vi "SPADQ_GetData.vi"(7 "DelayCorrect?":bool, 8 "error in (no error)":errorcluster, 11 "Digitizer Settings":T1 {"Trigger Settings"."Trig Slope" items=["Positive", "Negative"]; "Trigger Settings"."Level (mV)" format="%.2f"; "Trigger Settings"."Trig Coupling" items=["DC 1 MOhm", "AC 1 MOhm", "DC 50 Ohm", "AC 50 Ohm"]; "Trigger Settings"."Trig Source" items=["Chan 1", "External"]; "Rel Dig Delay" format="%.2f"; "DigTimeOut" format="%.2f"; "Avg Num" min=1; "Offset delay (us)" format="%.2f"; "Additional dig delay (us)" format="%.2f"; "Digitizer delay (us)" format="%.2f"}) -> (0 "error out":errorcluster, 1 "Data Out":i16[][](array[numeric]), 3 "ADQAPI Ref (out)":refnum<k24>)   [LabVIEW 2022 SP3]
doc: "_____AlazarTech, Scope_____\n\nSet the Trigger delay"
uses:
  C:/Windows/System32/ADQAPI_dotNet_helper.dll
  -DigitizerRoutines/DigitizerSettings.ctl
  -DigitizerRoutines/Digitizer.ctl
  -DigitizerRoutines/DigConfig.ctl
  -DigitizerRoutines/DigitizerID.ctl
  Memory.lvlib
panel:
  out "ADQ_ALL_CHANNELS_MASK":i32
  out "ADQ_GetNofChannels":u32
  in  "ChanMask":u8(ring)=1 items=["A"=1, "B"=2, "A&B"=3]
  in  "StartSample":u32
  out "return":i32
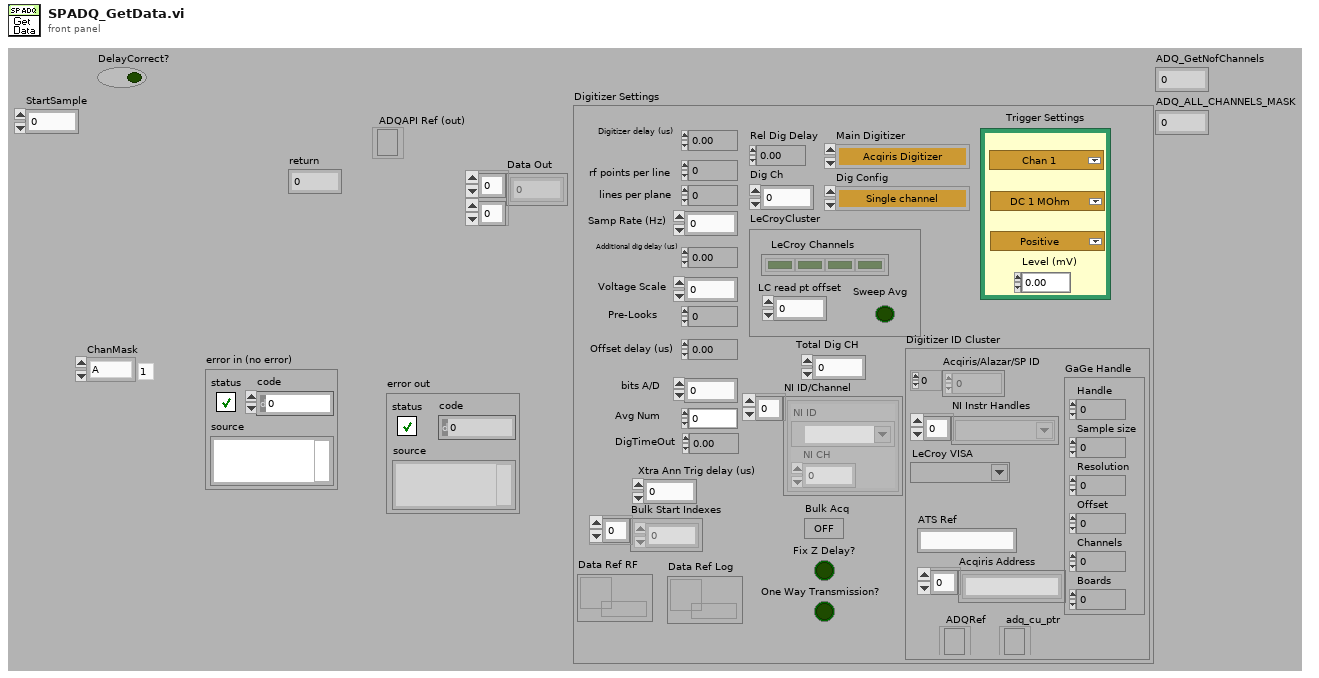
[diagram p1: front panel]
types:
  T1 = typedef "DigitizerSettings.ctl" = cluster{"Digitizer delay (us) ":dbl, "rf points per line":i32, "lines per plane":i32, "Samp Rate (Hz)":dbl, "Additional dig delay (us)":dbl, "Voltage Scale":dbl, "Pre-Looks":i32, "Offset delay (us)":dbl, "bits A/D":i8, "Avg Num":i32, "DigTimeOut":sgl, "Rel Dig Delay":sgl, "Dig Ch":i32, "LeCroyCluster":cluster{"LeCroy Channels":bool[], "LC read pt offset":dbl, "Sweep Avg":bool}, "Main Digitizer":T2, "Dig Config":T3, "Digitizer ID Cluster":T4, "Trigger Settings":cluster{"Trig Source":u16, "Trig Coupling":u16, "Trig Slope":u16, "Level (mV)":dbl}, "Bulk Acq":bool, "Bulk Start Indexes":i32[], "Data Ref RF":refnum<data-value>, "NI ID/Channel":cluster{"NI ID":refnum<k15>, "NI CH":i32}[], "Total Dig CH":i32, "Xtra Ann Trig delay (us)":dbl, "Fix Z Delay?":bool, "One Way Transmission?":bool, "Data Ref Log":refnum<data-value>}
  T2 = typedef "Digitizer.ctl" = enum16{"Acqiris Digitizer", "NI Digitizer", "LeCroy", "GaGe", "AlazarTech", "No Digitizer", "Teledyne"}
  T3 = typedef "DigConfig.ctl" = enum16{"Single channel", "2 Chans w/ 2 Acqiris", "2 Chans w/ 1 Acqiris", "5-CH Pulser New", "5-CH pulser w/ ann array", "5-pass style ann array", "Empty"}
  T4 = typedef "DigitizerID.ctl" = cluster{"Acqiris/Alazar/SP ID":u32[], "NI Instr Handles":refnum<k15>[], "LeCroy VISA":refnum<visa-resource-name>, "GaGe Handle":cluster{"Handle":u32, "Sample size":u32, "Resolution":i32, "Offset":i32, "Channels":u32, "Boards":u32}, "ATS Ref":string, "Acqiris Address":string[], "ADQRef":refnum<k24>, "adq_cu_ptr":refnum<k24>}
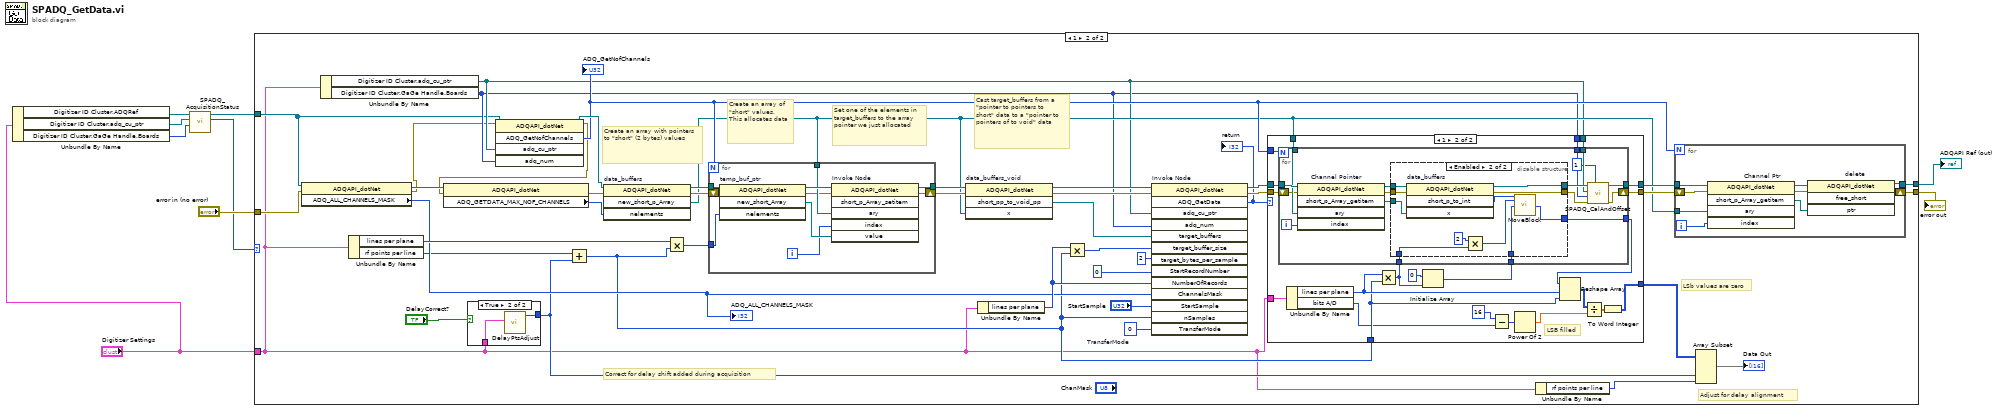
[diagram p0: block diagram]
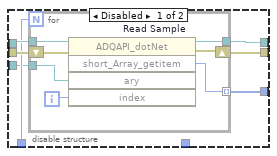
[diagram p5: hidden frame]
diagram:
  n1 = Unbundle By Name("Digitizer Settings") -> ("Digitizer ID Cluster.ADQRef"=w5:refnum<k24>, "Digitizer ID Cluster.adq_cu_ptr"=w4:refnum<k24>, "Digitizer ID Cluster.GaGe Handle.Boards"=w3:u32)
  n2 = call "SPADQ_AcquisitionStatus.vi"("adq_num"=w3, "adq_cu_ptr in"=w4, "ADQAPI Ref"=w5) -> ("return"=w6:i32, "ADQAPI Ref (out)"=w1:refnum<k24>)  [unwired: 5 in, 2 out]
  n3 = case shown="1" w6 {
    tunnel: [w11 w43] -> w9
    tunnel: [w10 w42] -> w8
    tunnel: "Digitizer Settings" -> [_ w13]
    tunnel: "error in (no error)" -> [w11 w22]
    tunnel: w1 -> [w10 w21]
    frame 0, Default {
    }
    frame 1 {
      w51 = u8 0  # TransferMode
      # "Adjust for delay alignment"
      # "LSb values are zero"
      # "Correct for delay shift added during acquisition"
      # "Cast target_buffers from a \"pointer to pointers to short\" data to a \"pointer to pointers of to void\" data"
      # "Create an array with pointers to \"short\" (2 bytes) values"
      # "Create an array of \"short\" values. This allocates data"
      # "Set one of the elements in target_buffers to the array pointer we just allocated"
      n4 = property class="ADQAPI_dotNet"(reference=w21, error in=w22) -> (reference out=w23:refnum<k24>, error out=w20:errorcluster, "ADQ_ALL_CHANNELS_MASK"=w28:i32)
      "ADQ_ALL_CHANNELS_MASK" <- w28
      n5 = Unbundle By Name(w13) -> ("Digitizer ID Cluster.adq_cu_ptr"=w26:refnum<k24>, "Digitizer ID Cluster.GaGe Handle.Boards"=w25:u32)
      n6 = Unbundle By Name(w13) -> ("lines per plane"=w45:i32, "rf points per line"=w24:i32)
      n7 = case shown="True" "DelayCorrect?" {
        tunnel: w13 -> [_ w56]
        tunnel: [_ w55] -> w16
        frame False {
        }
        frame True {
          n8 = call "DelayPtsAdjust.vi"("Digitizer Settings"=w56) -> ("PostDelayCorrection"=w55:u32)  [unwired: 9 in, 1 out]
        }
      }
      n9 = invoke class="ADQAPI_dotNet" method="ADQ_GetNofChannels"(reference=w21, error in=w20, "adq_cu_ptr"=w26, "adq_num"=w25) -> (reference out=w35:refnum<k24>, error out=w19:errorcluster, "ADQ_GetNofChannels"=w30:u32)  [unwired: 1 in, 2 out]
      "ADQ_GetNofChannels" <- w30
      n10 = property class="ADQAPI_dotNet"(reference=w23, error in=w19) -> (error out=w41:errorcluster, "ADQ_GETDATA_MAX_NOF_CHANNELS"=w29:i32)  [unwired: 1 out]
      n11 = Add(x=w24, y=w16) -> (x+y=w14:u32)
      n12 = invoke on="data_buffers" class="ADQAPI_dotNet" method="new_short_p_Array"(reference=w35, error in=w41, "nelements"=w29) -> (reference out=w50:refnum<k24>, error out=w40:errorcluster, "new_short_p_Array"=w27:refnum<k24>)  [unwired: 1 in, 1 out]
      n13 = Multiply(x=w45, y=w14) -> (x*y=w34:u32)
      n14 = for {
        N: w30 -> [_]
        tunnel: w27 -> [w137]
        tunnel: w34 -> [w136]
        shift-right: [w133] -> w39
        shift-left: w40 -> [w135]
        tunnel: w50 -> [w141]
        tunnel: [w138] -> w49
        i -> [w132]
        n15 = invoke on="temp_buf_ptr" class="ADQAPI_dotNet" method="new_short_Array"(reference=w141, error in=w135, "nelements"=w136) -> (reference out=w140:refnum<k24>, error out=w134:errorcluster, "new_short_Array"=w139:refnum<k24>)  [unwired: 1 in, 1 out]
        n16 = invoke on="Invoke Node" class="ADQAPI_dotNet" method="short_p_Array_setitem"(reference=w140, error in=w134, "ary"=w137, "index"=w132, "value"=w139) -> (reference out=w138:refnum<k24>, error out=w133:errorcluster)  [unwired: 1 in, 4 out]
      }
      n17 = invoke on="data_buffers_void" class="ADQAPI_dotNet" method="short_pp_to_void_pp"(reference=w49, error in=w39, "x"=w27) -> (reference out=w48:refnum<k24>, error out=w38:errorcluster, "short_pp_to_void_pp"=w44:refnum<k24>)  [unwired: 1 in, 1 out]
      n18 = Unbundle By Name(w13) -> ("lines per plane"=w33:i32)
      n19 = Multiply(x=w33, y=w14) -> (x*y=w32:u32)
      n20 = invoke on="Invoke Node" class="ADQAPI_dotNet" method="ADQ_GetData"(reference=w48, error in=w38, "adq_cu_ptr"=w26, "adq_num"=w25, "target_buffers"=w44, "target_buffer_size"=w32, "target_bytes_per_sample"=u8 2, "StartRecordNumber"=u32 0, "NumberOfRecords"=w33, "ChannelsMask"=w28, "StartSample"="StartSample", "nSamples"=w14, "TransferMode"=w51) -> (reference out=w47:refnum<k24>, error out=w37:errorcluster, "ADQ_GetData"=w31:i32)  [unwired: 1 in, 11 out]
      "return" <- w31
      n21 = case shown="1" w31 {
        tunnel: w47 -> [w58 w80]
        tunnel: w27 -> [_ w79]
        tunnel: [w58 w78] -> w46
        tunnel: w37 -> [w57 w77]
        tunnel: [w57 w76] -> w36
        tunnel: w30 -> [_ w75]
        tunnel: w13 -> [_ w72]
        tunnel: [_ w66] -> w18
        tunnel: w26 -> [_ w71]
        tunnel: w25 -> [_ w70]
        tunnel: w14 -> [_ w69]
        frame 0, Default {
        }
        frame 1 {
          # "LSB filled"
          n22 = Unbundle By Name(w72) -> ("lines per plane"=w73:i32, "bits A/D"=w59:i8)
          n23 = Multiply(x=w73, y=w69) -> (x*y=w61:u32)
          n24 = Initialize Array(i16 0, w61) -> (w60:i16[])
          n25 = for {
            N: w75 -> [_]
            tunnel: w79 -> [w96]
            tunnel: [w94] -> w74
            tunnel: w61 -> [w91]
            shift-right: [w86] -> w76
            shift-left: w77 -> [w93]
            tunnel: w80 -> [w97]
            tunnel: [w89] -> w78
            tunnel: w71 -> [w85]
            tunnel: w70 -> [w84]
            tunnel: w60 -> [w82]
            i -> [w88]
            n26 = invoke on="Channel Pointer" class="ADQAPI_dotNet" method="short_p_Array_getitem"(reference=w97, error in=w93, "ary"=w96, "index"=w88) -> (reference out=w95:refnum<k24>, error out=w92:errorcluster, "short_p_Array_getitem"=w83:refnum<k24>)  [unwired: 1 in, 2 out]
            n27 = disable-structure shown="Enabled" {
              disable-tunnel: w95 -> [w104 w117]
              disable-tunnel: [w103 w113] -> w94
              disable-tunnel: w92 -> [w102 w116]
              disable-tunnel: w91 -> [w101 w121]
              disable-tunnel: [w100 w115] -> w90
              disable-tunnel: [w99 w114] -> w87
              disable-tunnel: w83 -> [w98 w118]
              disable-tunnel: w82 -> [_ w112]
              frame Disabled {
                n28 = for {
                  N: w101 -> [_]
                  tunnel: [w110] -> w103 mode=indexing
                  tunnel: w98 -> [w108]
                  shift-right: [w106] -> w99
                  shift-left: w102 -> [w107]
                  tunnel: w104 -> [w109]
                  tunnel: [w111] -> w100
                  i -> [w105]
                  n29 = invoke on="Read Sample" class="ADQAPI_dotNet" method="short_Array_getitem"(reference=w109, error in=w107, "ary"=w108, "index"=w105) -> (reference out=w111:refnum<k24>, error out=w106:errorcluster, "short_Array_getitem"=w110:i16)  [unwired: 1 in, 2 out]
                }
              }
              frame Enabled {
                n30 = invoke on="data_buffers" class="ADQAPI_dotNet" method="short_p_to_int"(reference=w117, error in=w116, "x"=w118) -> (reference out=w115:refnum<k24>, error out=w114:errorcluster, "short_p_to_int"=w119:i32)  [unwired: 1 in, 1 out]
                n31 = Multiply(x=i16 2, y=w121) -> (x*y=w120:u32)
                n32 = call "MoveBlock.vi"("srcPointer"=w119, "size"=w120, "destination"=w112) -> ("destination"=w113:i16[])  [unwired: 13 in, 3 out]
              }
            }
            n33 = call "SPADQ_CalAndOffset.vi"("Channel"=u8 1, "error in (no error)"=w87, "adq_num"=w84, "adq_cu_ptr in"=w85, "ADQAPI Ref"=w90) -> ("error out"=w86:errorcluster, "ADQAPI Ref (out)"=w89:refnum<k24>)  [unwired: 2 in, 3 out]
          }
          n34 = Subtract(x=i8 16, y=w59) -> (x-y=w64:i8)
          n35 = Power Of 2(x=w64) -> (2^x=w63:dbl)
          n36 = Reshape Array(w74, w73, w69) -> (w68:i16[][])
          n37 = Divide(x=w68, y=w63) -> (x/y=w67:dbl[][])
          n38 = To Word Integer(number=w67) -> (16bit integer=w66:i16[][])
        }
      }
      n39 = Unbundle By Name(w13) -> ("rf points per line"=w12:i32)
      n40 = for {
        N: w30 -> [_]
        tunnel: w27 -> [w130]
        shift-right: [w128] -> w43
        shift-left: w36 -> [w126]
        tunnel: w46 -> [w129]
        tunnel: [w127] -> w42
        i -> [w124]
        n41 = invoke on="Channel Ptr" class="ADQAPI_dotNet" method="short_p_Array_getitem"(reference=w129, error in=w126, "ary"=w130, "index"=w124) -> (reference out=w131:refnum<k24>, error out=w125:errorcluster, "short_p_Array_getitem"=w123:refnum<k24>)  [unwired: 1 in, 2 out]
        n42 = invoke on="delete" class="ADQAPI_dotNet" method="free_short"(reference=w131, error in=w125, "ptr"=w123) -> (reference out=w127:refnum<k24>, error out=w128:errorcluster)  [unwired: 1 in, 2 out]
      }
      n43 = Array Subset(array=w18, index (col)=w16, length (col)=w12) -> (→"Data Out":i16[][])  [unwired: 2 in]
    }
  }
  "error out" <- w9
  "ADQAPI Ref (out)" <- w8
